vi "fit_focus.vi"(8 "error in (no error)":errorcluster, 9 "num_measurements":i32, 10 "heights":dbl[](array[numeric]), 11 "focus_values":dbl[](array[numeric])) -> (0 "error out":errorcluster, 2 "error":dbl, 3 "focus height":dbl)   [LabVIEW 2011, in "gVision.lvlib"]
uses:
  gVision.lvlib
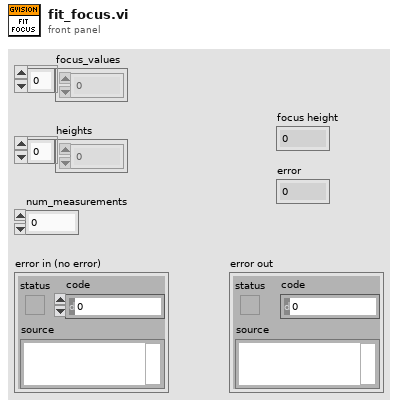
[diagram p1: front panel]
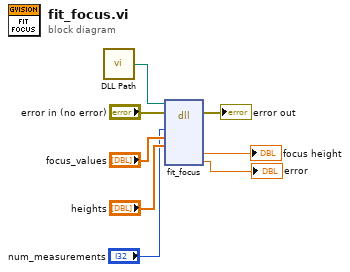
[diagram p0: block diagram]
diagram:
  n1 = call "DLL Path.vi"() -> ("DLL Path"=w3:path)  [unwired: 5 in]
  n2 = dll-call lib="?" fn="fit_focus"(path in=w3, error in="error in (no error)", "num_measurements"="num_measurements", "focus_values"="focus_values", "heights"="heights") -> (error out=→"error out":errorcluster, "mean"=→"focus height":dbl, "stdev"=→"error":dbl)  [unwired: 7 in, 1 out]
